vi "CPU Temperature.vi"(8 "error in (no error)":errorcluster, 11 "RP Communicator in":refnum<class "RP Communicator.lvclass">) -> (0 "error out":errorcluster, 2 "CPU Temperature":dbl, 3 "RP Communicator out":refnum<class "RP Communicator.lvclass">)   [LabVIEW 2016, in "RP Communicator.lvclass"]
uses:
  RP Communicator.lvclass
  RP Communicator.lvclass/RP Communicator.ctl
  RP Read Temperature TCP.vi
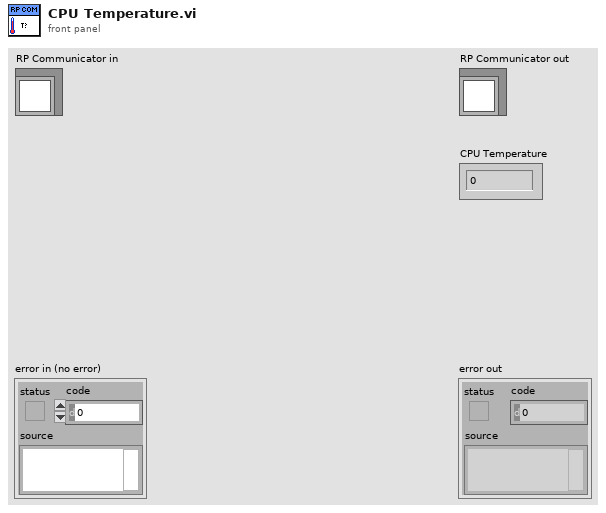
[diagram p1: front panel]
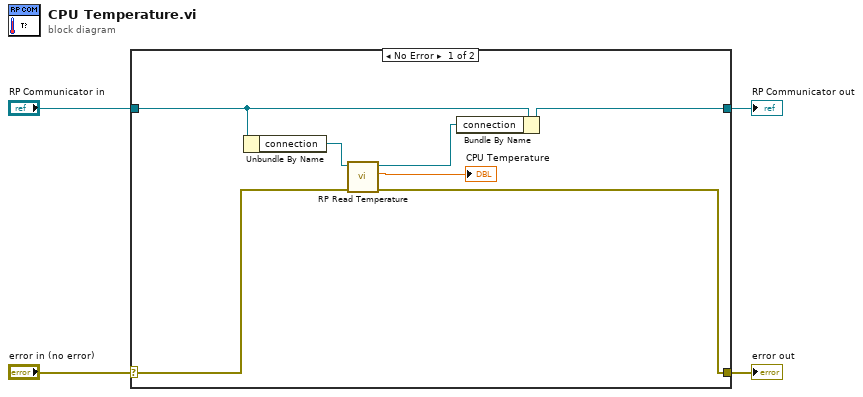
[diagram p0: block diagram]
diagram:
  n1 = case shown="No Error" "error in (no error)" {
    selector: "error in (no error)" -> [w9 w13]
    tunnel: [w8 w13] -> w3
    tunnel: [w7 w12] -> w1
    tunnel: "RP Communicator in" -> [w11 w12]
    frame No Error {
      n2 = Unbundle By Name(w11) -> ("connection"=w10:refnum<k5>)
      n3 = call-poly "RP Read Temperature.vi"("Error In"=w9, "connection ID"=w10) -> ("error out"=w8:errorcluster, "Thermometer"=→"CPU Temperature":dbl, "connection ID out"=w6:refnum<k5>)  [unwired: 7 in]
      n4 = Bundle By Name(cluster=w11, "connection"=w6) -> (w7:refnum<class "RP Communicator.lvclass">)
    }
    frame Error {
    }
  }
  "error out" <- w3
  "RP Communicator out" <- w1
